vi "STREAM_CREATE.vi"(2 "error in (no error)":errorcluster, 3 "Period":i32 min=0 max=65536, 4 "Channel":i8=2, 5 "VISA resource Input":refnum<visa-resource-name>) -> (0 "error out":errorcluster, 1 "VISA resource name out":refnum<visa-resource-name>)   [LabVIEW 2011]
panel:
  out "command sent":u8[](array[numeric])
  out "Read":u32
  out "Read Stream Create command":u8[](array[numeric])
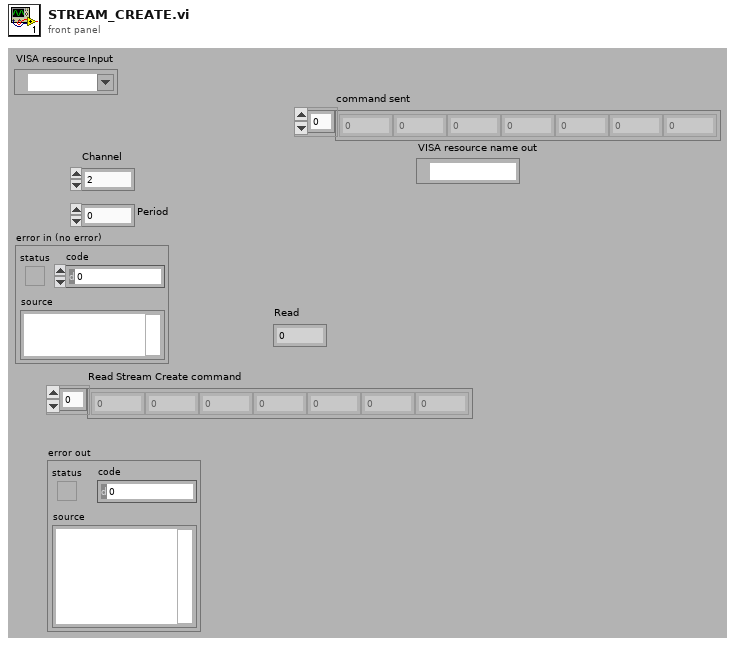
[diagram p1: front panel]
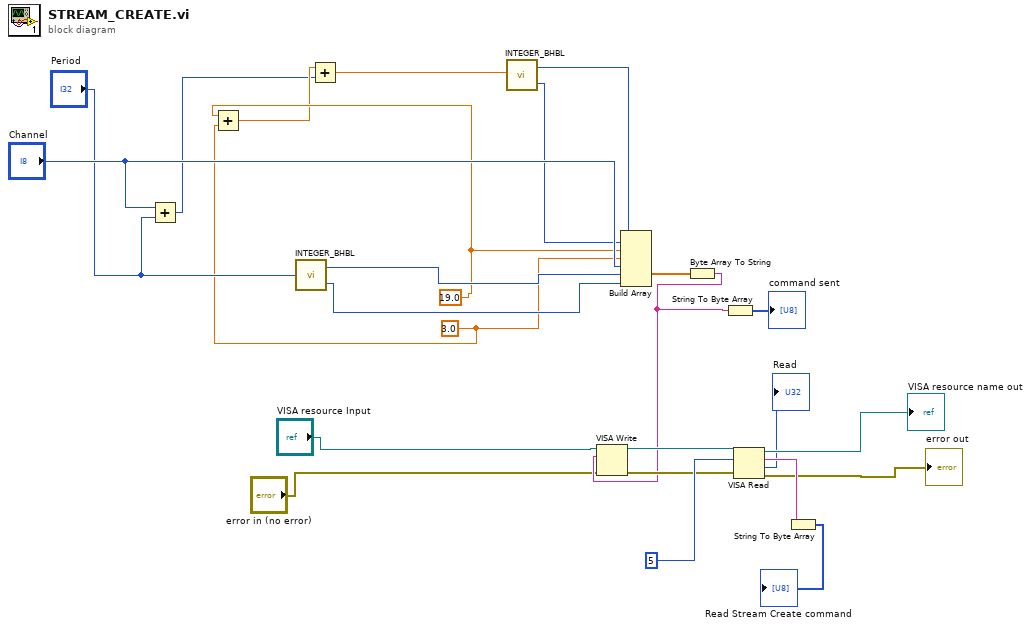
[diagram p0: block diagram]
diagram:
  w7 = 3.0 ("element")
  w6 = 19.0 ("element")
  n1 = Add(x="Channel", y="Period") -> (x+y=w4:i32)
  n2 = Add(x=w6, y=w7) -> (x+y=w5:dbl)
  n3 = call "INTEGER_BHBL.vi"("int16"="Period") -> ("Lvalue"=w14:u8, "HValue"=w13:u8)
  n4 = Add(x=w5, y=w4) -> (x+y=w3:dbl)
  n5 = call "INTEGER_BHBL.vi"("int16"=w3) -> ("Lvalue"=w1:u8, "HValue"=w2:u8)
  n6 = Build Array(w2, w1, w6, w7, "Channel", w13, w14) -> (w19:dbl[])
  n7 = Byte Array To String(unsigned byte array=w19) -> (string=w16:string)
  n8 = VISA Write(VISA resource name="VISA resource Input", write buffer=w16, error in (no error)="error in (no error)") -> (VISA resource name out=w20:refnum<visa-resource-name>, error out=w21:errorcluster)  [unwired: 1 out]
  n9 = String To Byte Array(string=w16) -> (unsigned byte array=→"command sent":u8[])
  n10 = VISA Read(VISA resource name=w20, byte count=u32 5, error in (no error)=w21) -> (VISA resource name out=→"VISA resource name out":refnum<visa-resource-name>, read buffer=w23:string, return count=→"Read":u32, error out=→"error out":errorcluster)
  n11 = String To Byte Array(string=w23) -> (unsigned byte array=→"Read Stream Create command":u8[])
